vi "optimization_testing.vi"() -> (3 "Optimized Location":dbl[](array[numeric]), 10 "yStart":dbl=123.0 format="%#_13g", 11 "xStart":dbl=264.0 format="%#_13g")   [LabVIEW 2024]
uses:
  <vilib>/numeric/Random Number (Range) DBL.vi
  0b4b40c4-ef97-49a3-bff4-9c7e9883bc37.vi
  5b59031f-b1ff-41af-80a7-e72a33ebffa1.vi
  <vilib>/Array/Sort 2D Array - Pop Stack.vi
  <vilib>/Array/Sort 2D Array - Push Stack.vi
  0b4b40c4-ef97-49a3-bff4-9c7e9883bc37.vi/269d4b3b-47f5-49e3-8884-44851e4dd9d5.vi
  0b4b40c4-ef97-49a3-bff4-9c7e9883bc37.vi/6d99389c-673d-4efb-bf33-19b32bcf4cf8.vi
  5b59031f-b1ff-41af-80a7-e72a33ebffa1.vi/269d4b3b-47f5-49e3-8884-44851e4dd9d5.vi
  5b59031f-b1ff-41af-80a7-e72a33ebffa1.vi/6d99389c-673d-4efb-bf33-19b32bcf4cf8.vi
  <vilib>/Analysis/NI_AALBase.lvlib
panel:
  out "Array":dbl[](array[numeric])
  out "elapsed time (s)":dbl
  out "n":i32(slide) scale=0.0..1.0
  out "GrAsc - avgs":dbl[][](array[numeric])
  out "NM - avgs":dbl[][](array[numeric])
  in  "nTrials":i32=1000
  out "std dev of simplex values 2":dbl
  out "simplex leg lengths 2":dbl[](array[numeric])
  out "iterations timeout 2":bool
  out "simplex converge 2":bool
  out "value converge 2":bool
  out "Starting Points":dbl[][][](array[numeric])
  in  "k":dbl=50.0
  out "GrAsc res":dbl[](array[numeric])
  out "x_c":dbl[](array[numeric])
  out "x_e":dbl[](array[numeric])
  out "x_r":dbl[](array[numeric])
  out "x_o":dbl[](array[numeric])
  out "iterations timeout":bool
  out "simplex converge":bool
  out "value converge":bool
  out "simplex leg lengths":dbl[](array[numeric])
  out "std dev of simplex values":dbl
  in  "stop":bool
  # "Avg"
  # "Std Dev"
  # "X"
  # "Y"
  # "Value"
  # "n Trials"
  # "Failures"
  # "Avg"
  # "Std Dev"
  # "X"
  # "Y"
  # "Value"
  # "n Trials"
  # "Failures"
  # "centroid"
  # "reflection point"
  # "expansion point"
  # "contraction point"
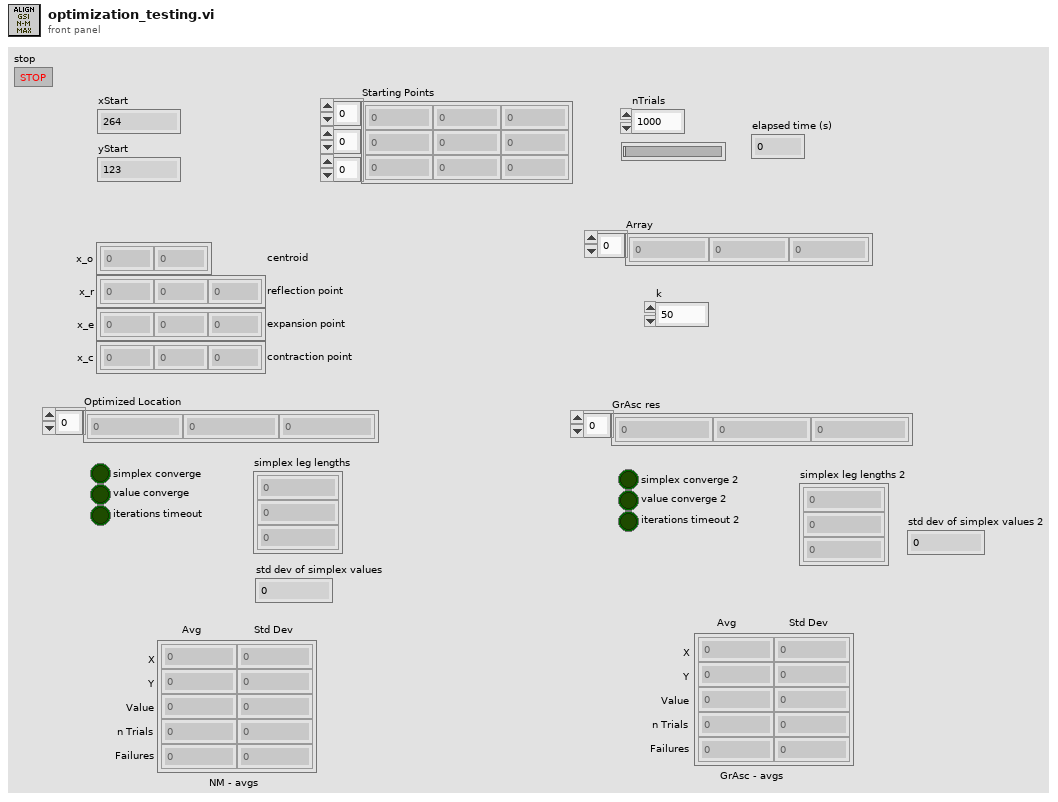
[diagram p1: front panel]
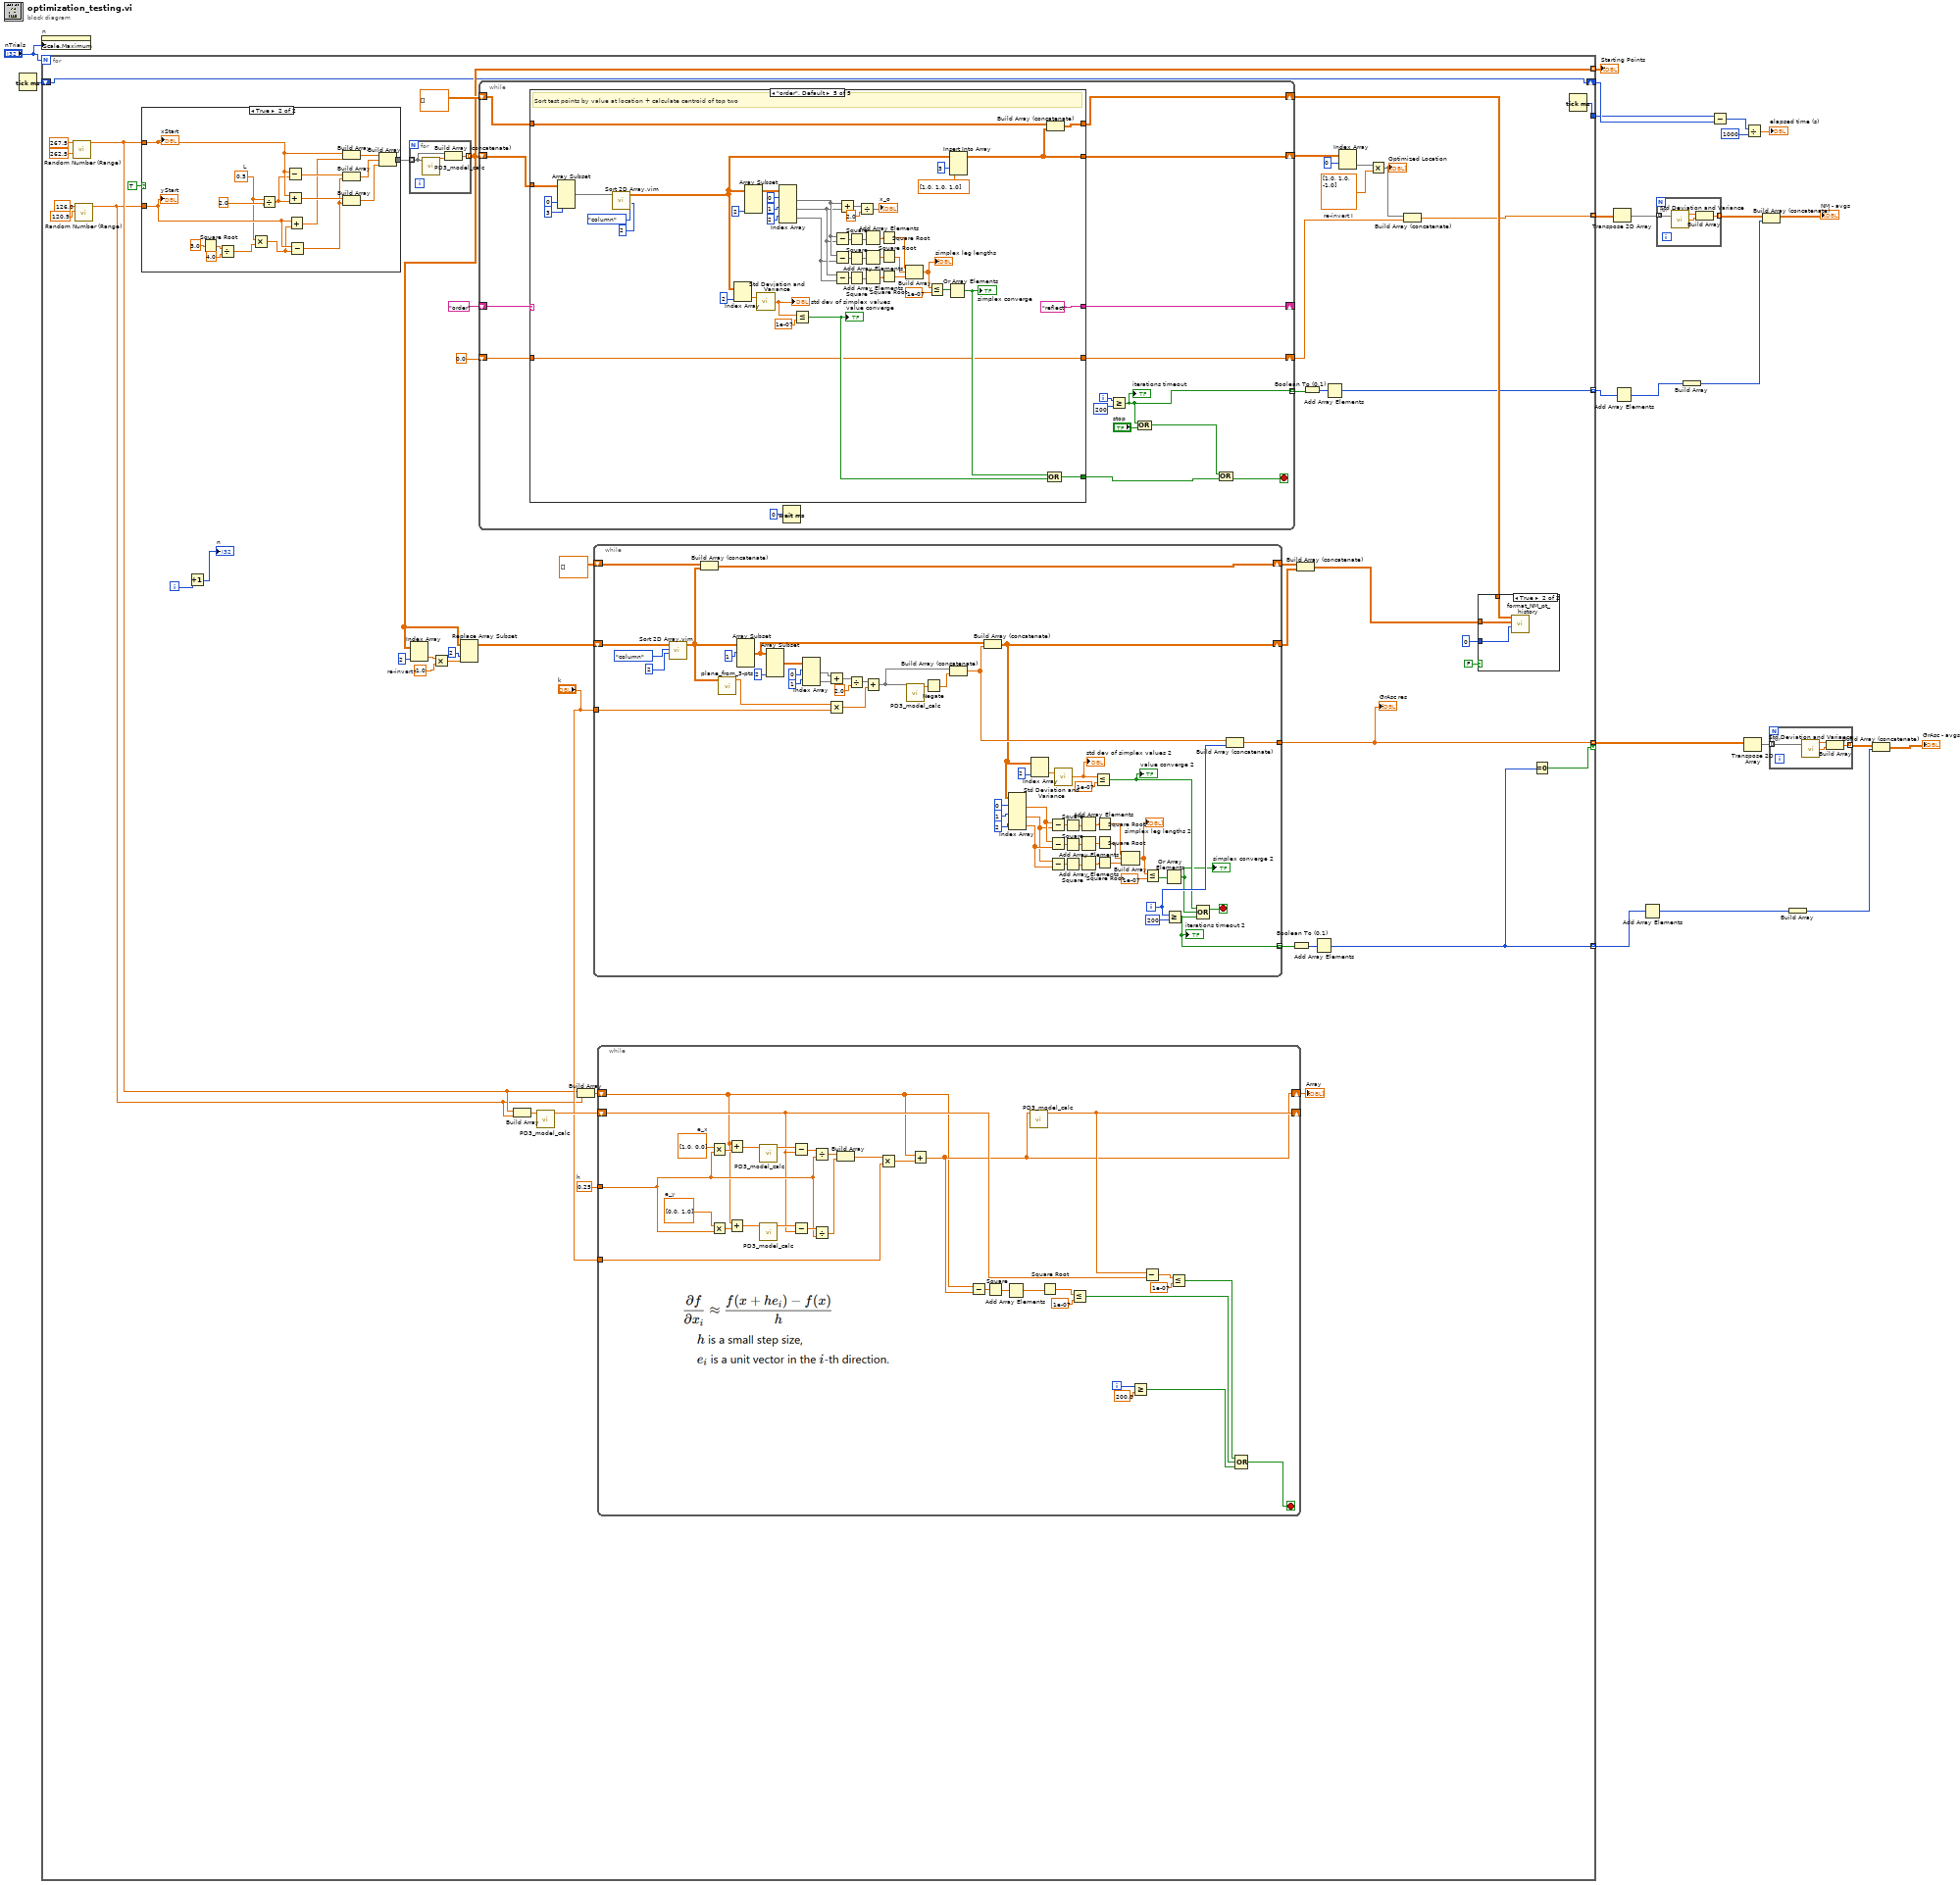
[diagram p0: block diagram]
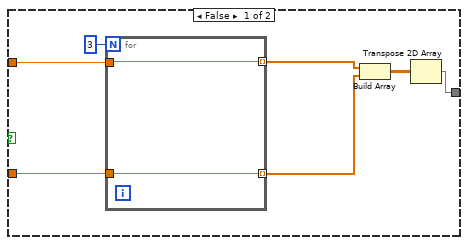
[diagram p3: hidden frame]
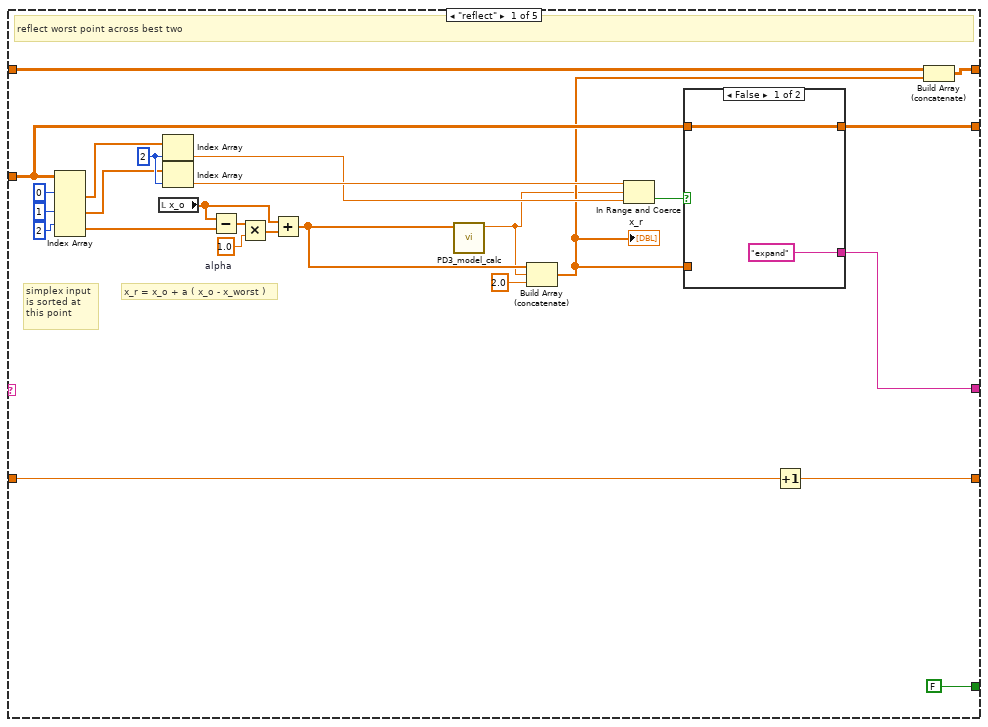
[diagram p4: hidden frame]
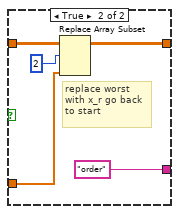
[diagram p5: hidden frame]
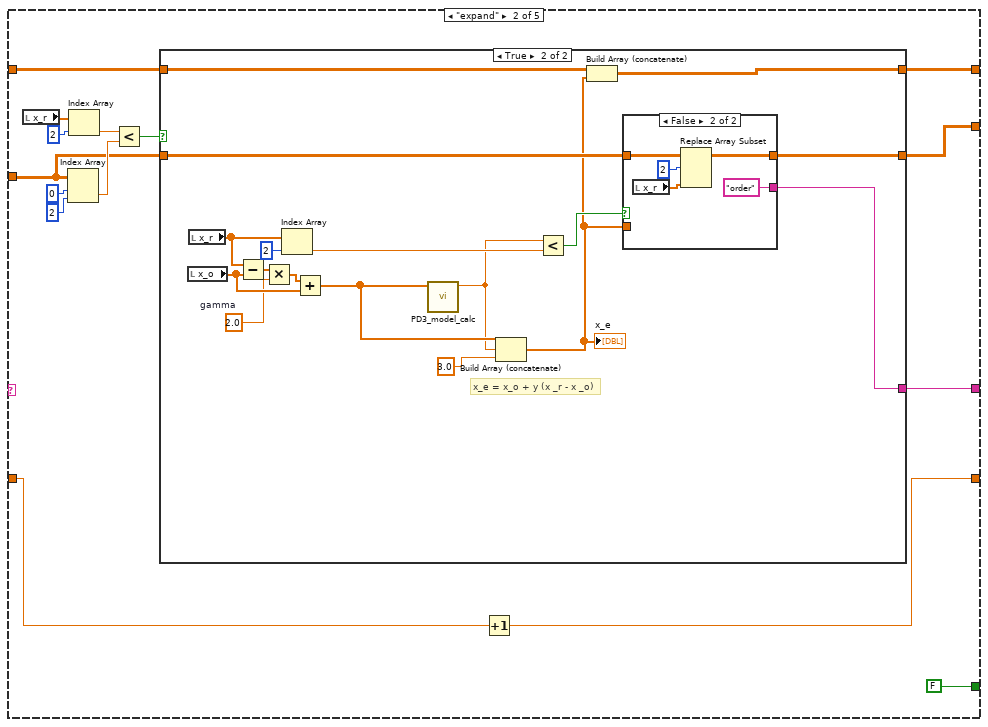
[diagram p6: hidden frame]
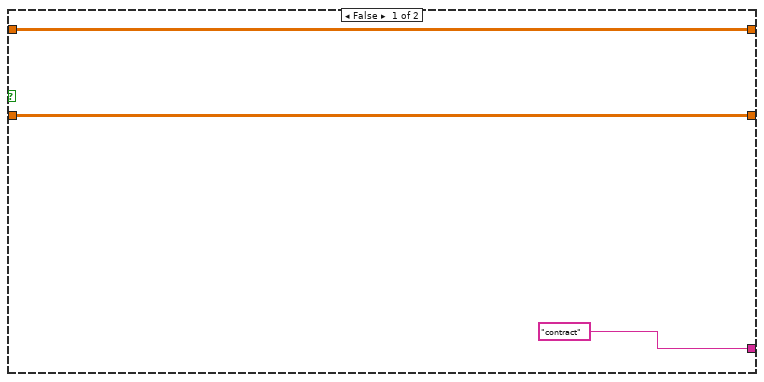
[diagram p7: hidden frame]
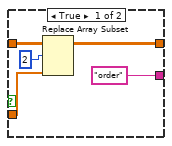
[diagram p8: hidden frame]
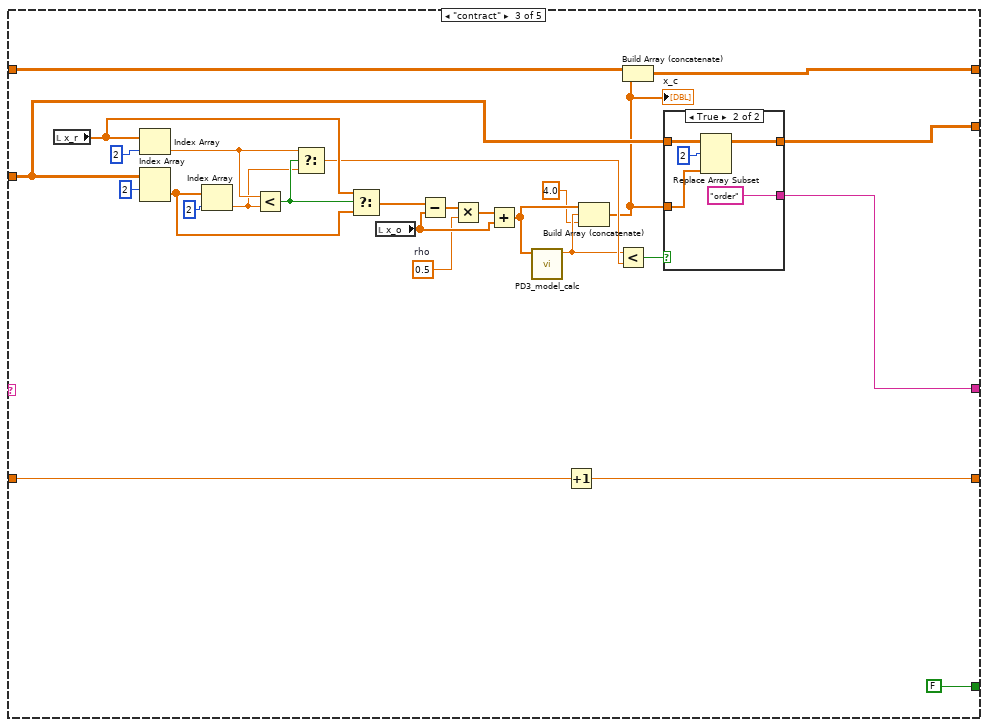
[diagram p9: hidden frame]
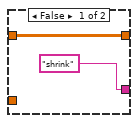
[diagram p10: hidden frame]
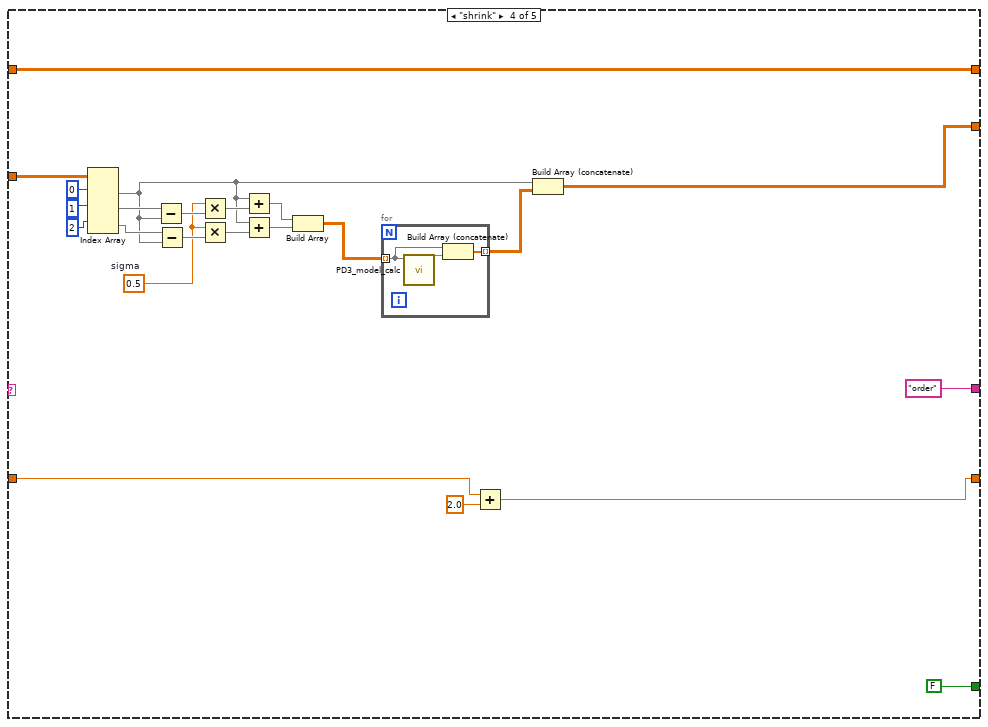
[diagram p11: hidden frame]
diagram:
  n1 = Tick Count (ms)() -> (millisecond timer value=w4:u32)
  n2 = property on="n" class="Slide (strict)"("Scale.Maximum"="nTrials") -> ()  [unwired: 2 in, 2 out]
  n3 = for {
    N: "nTrials" -> [_]
    tunnel: [w47] -> w21 mode=indexing
    tunnel: [w45] -> w20 mode=indexing
    tunnel: [w42] -> w15 mode=indexing if=w39
    tunnel: [w38] -> w14 mode=indexing
    tunnel: [w35] -> w10 mode=indexing
    shift-right: [w32] -> w3
    shift-left: w4 -> [w32]
    tunnel: [w31] -> w1
    i -> [w34]
    w28 = 0.25  # h
    w60 = -1.0  # re-invert I
    w67 = dbl[] [1.0, 1.0, -1.0]  # re-invert I
    n4 = call-poly <vilib>:"Random Number (Range).vi"("lower bound (0)"=262.5, "upper bound (100)"=267.5) -> ("number"=w26:dbl)  [unwired: 9 in]
    n5 = call-poly <vilib>:"Random Number (Range).vi"("lower bound (0)"=120.9 ("upper bound (100)"), "upper bound (100)"=126.0 ("lower bound (0)")) -> ("number"=w25:dbl)  [unwired: 9 in]
    n6 = case shown="True" TRUE {
      tunnel: [w109 w132] -> w55
      tunnel: w26 -> [w114 w124]
      tunnel: w25 -> [w113 w123]
      frame False {
        n7 = for {
          N: 3 -> [_]
          tunnel: w114 -> [w117]
          tunnel: [w117] -> w112 mode=indexing
          tunnel: w113 -> [w116]
          tunnel: [w116] -> w110 mode=indexing
        }
        n8 = Build Array(w112, w110) -> (w111:dbl[][])
        n9 = Transpose 2D Array(2D array=w111) -> (transposed array=w109:dbl[][])
      }
      frame True {
        w118 = 0.5  # L
        n10 = Square Root(x=3.0) -> (sqrt(x)=w131:dbl)
        n11 = Divide(x=w131, y=4.0) -> (x/y=w120:dbl)
        n12 = Multiply(x=w118, y=w120) -> (x*y=w119:dbl)
        n13 = Divide(x=w118, y=2.0) -> (x/y=w121:dbl)
        n14 = Subtract(x=w124, y=w121) -> (x-y=w128:dbl)
        n15 = Add(x=w124, y=w121) -> (x+y=w127:dbl)
        n16 = Add(x=w123, y=w119) -> (x+y=w126:dbl)
        n17 = Subtract(x=w123, y=w119) -> (x-y=w125:dbl)
        n18 = Build Array(w124, w126) -> (w133:dbl[])
        n19 = Build Array(w128, w125) -> (w134:dbl[])
        n20 = Build Array(w127, w125) -> (w135:dbl[])
        n21 = Build Array(w133, w134, w135) -> (w132:dbl[][])
        "xStart" <- w124
        "yStart" <- w123
      }
    }
    n22 = Increment(x=w34) -> (x+1=→"n":i32)
    n23 = for {
      tunnel: w55 -> [w193] mode=indexing
      tunnel: [w195] -> w47 mode=indexing
      n24 = call "PD3_model_calc.vi"("pos_in"=w193) -> ("I_out"=w194:dbl)  [unwired: 10 in]
      n25 = Build Array (concatenate)(w193, w194) -> (w195:dbl[])
    }
    n26 = Index Array(array=w47, index (col)=2 ("disabled index (col)")) -> (element=w58:dbl[])  [unwired: 1 in]
    n27 = Multiply(x=w58, y=w60) -> (x*y=w56:dbl[])
    n28 = Replace Array Subset(array=w47, new element=w56, index (col)=2 ("disabled index (col)")) -> (w54:dbl[][])  [unwired: 1 in]
    n29 = while {
      shift-right: [w209] -> w72
      shift-left: w47 -> [w207]
      shift-right: [w210] -> _
      shift-left: "order" -> [w211]
      shift-right: [w205] -> w66
      shift-left: dbl[][] [] -> [w206]
      shift-right: [w199] -> w43
      shift-left: 0.0 -> [w200]
      tunnel: [w198] -> w36 mode=indexing
      i -> [w201]
      stop <- w197 stop-if-true
      n30 = case shown="\"order\", Default" w211 {
        tunnel: w207 -> [w222 w252 w302 w345 w388]
        tunnel: [FALSE FALSE FALSE FALSE w364] -> w203
        tunnel: [w221 w251 w303 w334 w353] -> w209
        tunnel: [w223 w250 w304 "order" "reflect"] -> w210
        tunnel: w206 -> [w219 w248 w298 w332 w352]
        tunnel: [w218 w247 w295 w332 w358] -> w205
        tunnel: w200 -> [w213 w246 w291 w326 w350]
        tunnel: [w212 w245 w290 w325 w350] -> w199
        frame "reflect" {
          w214 = 1.0  # alpha
          w231 = 2 ("index")
          # "simplex input\nis sorted at\nthis point"
          # "x_r = x_o + a ( x_o - x_worst )"
          # "reflect worst point across best two"
          n31 = Index Array(array=w222, index (row) #1=0 ("index (row)"), index (row) #2=1 ("index (row)"), index (row) #3=2 ("index (row)")) -> (element #1=w230:dbl[], element #2=w229:dbl[], element #3=w232:dbl[])  [unwired: 3 in]
          n32 = local read "x_o"() -> (w224:dbl[])
          n33 = Index Array(array=w230, index=w231) -> (element=w227:dbl)
          n34 = Index Array(array=w229, index=w231) -> (element=w228:dbl)
          n35 = Subtract(x=w224, y=w232) -> (x-y=w236:dbl[])
          n36 = Multiply(x=w236, y=w214) -> (x*y=w235:dbl[])
          n37 = Add(x=w224, y=w235) -> (x+y=w225:dbl[])
          n38 = call "PD3_model_calc.vi"("pos_in"=w225) -> ("I_out"=w216:dbl)  [unwired: 10 in]
          n39 = Build Array (concatenate)(w225, w216, 2.0) -> (w217:dbl[])
          "x_r" <- w217
          n40 = In Range and Coerce(upper limit=w228, x=w216, lower limit=w227) -> (In Range?=w226:bool)  [unwired: 1 out]
          n41 = case shown="False" w226 {
            tunnel: ["expand" "order"] -> w223
            tunnel: w222 -> [w238 w244]
            tunnel: [w238 w241] -> w221
            tunnel: w217 -> [_ w242]
            frame False {
            }
            frame True {
              # "replace worst \nwith x_r go back\nto start"
              n42 = Replace Array Subset(array=w244, new element=w242, index (row)=2) -> (w241:dbl[][])  [unwired: 1 in]
            }
          }
          n43 = Increment(x=w213) -> (x+1=w212:dbl)
          n44 = Build Array (concatenate)(w219, w217) -> (w218:dbl[][])
        }
        frame "expand" {
          n45 = local read "x_r"() -> (w257:dbl[])
          n46 = Index Array(array=w252, index (row)=0, index (col)=2 ("disabled index (col)")) -> (element=w255:dbl)
          n47 = Index Array(array=w257, index=2) -> (element=w254:dbl)
          n48 = Less?(x=w254, y=w255) -> (x < y?=w253:bool)
          n49 = case shown="True" w253 {
            tunnel: w252 -> [w262 w272]
            tunnel: [w262 w270] -> w251
            tunnel: ["contract" w269] -> w250
            tunnel: w248 -> [w260 w267]
            tunnel: [w260 w266] -> w247
            frame False {
            }
            frame True {
              w263 = 2.0  # gamma
              # "x_e = x_o + y (x _r - x _o)"
              n50 = local read "x_o"() -> (w277:dbl[])
              n51 = local read "x_r"() -> (w276:dbl[])
              n52 = Subtract(x=w276, y=w277) -> (x-y=w279:dbl[])
              n53 = Multiply(x=w279, y=w263) -> (x*y=w278:dbl[])
              n54 = Index Array(array=w276, index=2) -> (element=w274:dbl)
              n55 = Add(x=w278, y=w277) -> (x+y=w271:dbl[])
              n56 = call "PD3_model_calc.vi"("pos_in"=w271) -> ("I_out"=w268:dbl)  [unwired: 10 in]
              n57 = Build Array (concatenate)(w271, w268, 3.0) -> (w265:dbl[])
              "x_e" <- w265
              n58 = Less?(x=w268, y=w274) -> (x < y?=w273:bool)
              n59 = Build Array (concatenate)(w267, w265) -> (w266:dbl[][])
              n60 = case shown="False" w273 {
                tunnel: w272 -> [w283 w288]
                tunnel: w265 -> [w282 _]
                tunnel: [w281 w287] -> w270
                tunnel: ["order" "order"] -> w269
                frame True {
                  n61 = Replace Array Subset(array=w283, new element=w282, index (row)=2) -> (w281:dbl[][])  [unwired: 1 in]
                }
                frame False {
                  n62 = local read "x_r"() -> (w285:dbl[])
                  n63 = Replace Array Subset(array=w288, new element=w285, index (row)=2) -> (w287:dbl[][])  [unwired: 1 in]
                }
              }
            }
          }
          n64 = Increment(x=w246) -> (x+1=w245:dbl)
        }
        frame "contract" {
          w292 = 0.5  # rho
          n65 = local read "x_r"() -> (w313:dbl[])
          n66 = Index Array(array=w313, index=2) -> (element=w308:dbl)
          n67 = Index Array(array=w302, index (row)=2) -> (element=w312:dbl[])  [unwired: 1 in]
          n68 = Index Array(array=w312, index=2) -> (element=w307:dbl)
          n69 = Less?(x=w308, y=w307) -> (x < y?=w309:bool)
          n70 = Select(t=w308, s=w309, f=w307) -> (s? t:f=w306:dbl)
          n71 = Select(t=w313, s=w309, f=w312) -> (s? t:f=w311:dbl[])
          n72 = local read "x_o"() -> (w300:dbl[])
          n73 = Subtract(x=w311, y=w300) -> (x-y=w310:dbl[])
          n74 = Multiply(x=w310, y=w292) -> (x*y=w301:dbl[])
          n75 = Add(x=w301, y=w300) -> (x+y=w297:dbl[])
          n76 = call "PD3_model_calc.vi"("pos_in"=w297) -> ("I_out"=w296:dbl)  [unwired: 10 in]
          n77 = Increment(x=w291) -> (x+1=w290:dbl)
          n78 = Build Array (concatenate)(w297, w296, 4.0 ("array")) -> (w294:dbl[])
          "x_c" <- w294
          n79 = Less?(x=w296, y=w306) -> (x < y?=w305:bool)
          n80 = Build Array (concatenate)(w298, w294) -> (w295:dbl[][])
          n81 = case shown="True" w305 {
            tunnel: ["shrink" "order"] -> w304
            tunnel: [w317 w319] -> w303
            tunnel: w302 -> [w317 w321]
            tunnel: w294 -> [_ w320]
            frame False {
            }
            frame True {
              n82 = Replace Array Subset(array=w321, new element=w320, index (row)=2) -> (w319:dbl[][])  [unwired: 1 in]
            }
          }
        }
        frame "shrink" {
          w331 = 0.5  # sigma
          n83 = Index Array(array=w345, index (row) #1=0 ("index (row)"), index (row) #2=1 ("index (row)"), index (row) #3=2 ("index (row)")) -> (element #1=w335:dbl[], element #2=w341:dbl[], element #3=w340:dbl[])  [unwired: 3 in]
          n84 = Subtract(x=w341, y=w335) -> (x-y=w338:dbl[])
          n85 = Subtract(x=w340, y=w335) -> (x-y=w339:dbl[])
          n86 = Multiply(x=w331, y=w338) -> (x*y=w337:dbl[])
          n87 = Multiply(x=w331, y=w339) -> (x*y=w336:dbl[])
          n88 = Add(x=w335, y=w337) -> (x+y=w330:dbl[])
          n89 = Add(x=w335, y=w336) -> (x+y=w329:dbl[])
          n90 = Build Array(w330, w329) -> (w328:dbl[][])
          n91 = for {
            tunnel: w328 -> [w347] mode=indexing
            tunnel: [w349] -> w327 mode=indexing
            n92 = call "PD3_model_calc.vi"("pos_in"=w347) -> ("I_out"=w348:dbl)  [unwired: 10 in]
            n93 = Build Array (concatenate)(w347, w348) -> (w349:dbl[])
          }
          n94 = Add(x=w326, y=2.0) -> (x+y=w325:dbl)
          n95 = Build Array (concatenate)(w335, w327) -> (w334:dbl[][])
        }
        frame "order", Default {
          # "Sort test points by value at location + calculate centroid of top two"
          n96 = Array Subset(array=w388, index (col)=0 ("index"), length (col)=3 ("length")) -> (w351:dbl[][])  [unwired: 2 in]
          n97 = call "Sort 2D Array.vim"("index"=2, "dimension to index (column)"=enum16{"column", "row"}."column", "2D array"=w351) -> ("sorted 2D array"=w356:dbl[][])  [unwired: 7 in, 1 out]
          n98 = Index Array(array=w356, index (col)=2 ("index")) -> (element=w382:dbl[])  [unwired: 1 in]
          n99 = Array Subset(array=w356, length (col)=2 ("length")) -> (w381:dbl[][])  [unwired: 3 in]
          n100 = call <vilib>:"Std Deviation and Variance.vi"("X"=w382) -> ("standard deviation"=w357:dbl)  [unwired: 1 in, 2 out]
          "std dev of simplex values" <- w357
          n101 = Index Array(array=w381, index (row) #1=0 ("index (row)"), index (row) #2=1 ("index (row)"), index (row) #3=2 ("index (row)")) -> (element #1=w361:dbl[], element #2=w360:dbl[], element #3=w359:dbl[])  [unwired: 3 in]
          n102 = Less Or Equal?(x=w357, y=1e-07) -> (x <= y?=w363:bool)
          "value converge" <- w363
          n103 = Subtract(x=w361, y=w360) -> (x-y=w379:dbl[])
          n104 = Subtract(x=w361, y=w359) -> (x-y=w371:dbl[])
          n105 = Subtract(x=w360, y=w359) -> (x-y=w374:dbl[])
          n106 = Add(x=w361, y=w360) -> (x+y=w386:dbl[])
          n107 = Square(x=w379) -> (x^2=w378:dbl[])
          n108 = Square(x=w371) -> (x^2=w375:dbl[])
          n109 = Square(x=w374) -> (x^2=w373:dbl[])
          n110 = Divide(x=w386, y=2.0) -> (x/y=→"x_o":dbl[])
          n111 = Add Array Elements(numeric array=w378) -> (sum=w377:dbl)
          n112 = Add Array Elements(numeric array=w375) -> (sum=w376:dbl)
          n113 = Add Array Elements(numeric array=w373) -> (sum=w372:dbl)
          n114 = Square Root(x=w377) -> (sqrt(x)=w368:dbl)
          n115 = Square Root(x=w376) -> (sqrt(x)=w369:dbl)
          n116 = Square Root(x=w372) -> (sqrt(x)=w370:dbl)
          n117 = Build Array(w368, w369, w370) -> (w367:dbl[])
          "simplex leg lengths" <- w367
          n118 = Less Or Equal?(x=w367, y=1e-07) -> (x <= y?=w365:bool[])
          n119 = Or Array Elements(Boolean array=w365) -> (logical OR=w362:bool)
          "simplex converge" <- w362
          n120 = Insert Into Array(array=w356, index (col)=3 ("disabled index (col)"), new element=dbl[] [1.0, 1.0, 1.0] ("new element/subarray")) -> (w353:dbl[][])  [unwired: 1 in]
          n121 = Build Array (concatenate)(w352, w353) -> (w358:dbl[][])
          n122 = Compound Arithmetic op=OR(w362, w363) -> (w364:bool)
        }
      }
      n123 = Wait (ms)(milliseconds to wait=u32 0) -> ()  [unwired: 1 out]
      n124 = Greater Or Equal?(x=w201, y=200) -> (x >= y?=w198:bool)
      "iterations timeout" <- w198
      n125 = Compound Arithmetic op=OR(w198, "stop") -> (w196:bool)
      n126 = Compound Arithmetic op=OR(w196, w203) -> (w197:bool)
    }
    n127 = Build Array(w26, w25) -> (w30:dbl[])
    n128 = call "PD3_model_calc.vi"("pos_in"=w30) -> ("I_out"=w29:dbl)  [unwired: 10 in]
    n129 = Build Array(w26, w25) -> (w24:dbl[])
    n130 = while {
      tunnel: "k" -> [w168]
      shift-right: [w171] -> w53
      shift-left: dbl[][] [] -> [w192]
      shift-right: [w149] -> w52
      shift-left: w54 -> [w189]
      tunnel: [w163] -> w42
      tunnel: [w136] -> w41 mode=indexing
      i -> [w162]
      stop <- w164 stop-if-true
      n131 = call "Sort 2D Array.vim"("index"=2, "dimension to index (column)"=enum16{"column", "row"}."column", "2D array"=w189) -> ("sorted 2D array"=w170:dbl[][])  [unwired: 7 in, 1 out]
      n132 = Build Array (concatenate)(w192, w170) -> (w171:dbl[][])
      n133 = call "plane_from_3-pts.vi"("Input"=w170) -> ("gradient-out"=w173:dbl[])  [unwired: 9 in, 1 out]
      n134 = Array Subset(array=w170, index (row)=1 ("index")) -> (w178:dbl[][])  [unwired: 3 in]
      n135 = Array Subset(array=w178, length (col)=2 ("length")) -> (w180:dbl[][])  [unwired: 3 in]
      n136 = Index Array(array=w180, index (row) #1=0 ("index (row)"), index (row) #2=1 ("index (row)")) -> (element #1=w185:dbl[], element #2=w184:dbl[])  [unwired: 2 in]
      n137 = Add(x=w185, y=w184) -> (x+y=w183:dbl[])
      n138 = Multiply(x=w173, y=w168) -> (x*y=w174:dbl[])
      n139 = Divide(x=w183, y=2.0) -> (x/y=w176:dbl[])
      n140 = Add(x=w176, y=w174) -> (x+y=w175:dbl[])
      n141 = call "PD3_model_calc.vi"("pos_in"=w175) -> ("I_out"=w179:dbl)  [unwired: 10 in]
      n142 = Negate(x=w179) -> (-x=w177:dbl)
      n143 = Build Array (concatenate)(w175, w177) -> (w169:dbl[])
      n144 = Build Array (concatenate)(w178, w169) -> (w149:dbl[][])
      n145 = Index Array(array=w149, index (row) #1=0 ("index (row)"), index (row) #2=1 ("index (row)"), index (row) #3=2 ("index (row)")) -> (element #1=w148:dbl[], element #2=w146:dbl[], element #3=w147:dbl[])  [unwired: 3 in]
      n146 = Index Array(array=w149, index (col)=2 ("index")) -> (element=w167:dbl[])  [unwired: 1 in]
      n147 = Subtract(x=w148, y=w146) -> (x-y=w150:dbl[])
      n148 = Subtract(x=w148, y=w147) -> (x-y=w158:dbl[])
      n149 = Subtract(x=w146, y=w147) -> (x-y=w155:dbl[])
      n150 = call <vilib>:"Std Deviation and Variance.vi"("X"=w167) -> ("standard deviation"=w137:dbl)  [unwired: 1 in, 2 out]
      "std dev of simplex values 2" <- w137
      n151 = Square(x=w150) -> (x^2=w151:dbl[])
      n152 = Square(x=w158) -> (x^2=w154:dbl[])
      n153 = Square(x=w155) -> (x^2=w156:dbl[])
      n154 = Add Array Elements(numeric array=w151) -> (sum=w152:dbl)
      n155 = Add Array Elements(numeric array=w154) -> (sum=w153:dbl)
      n156 = Add Array Elements(numeric array=w156) -> (sum=w157:dbl)
      n157 = Less Or Equal?(x=w137, y=1e-07) -> (x <= y?=w140:bool)
      "value converge 2" <- w140
      n158 = Square Root(x=w152) -> (sqrt(x)=w161:dbl)
      n159 = Square Root(x=w153) -> (sqrt(x)=w160:dbl)
      n160 = Square Root(x=w157) -> (sqrt(x)=w159:dbl)
      n161 = Build Array(w161, w160, w159) -> (w138:dbl[])
      "simplex leg lengths 2" <- w138
      n162 = Less Or Equal?(x=w138, y=1e-07) -> (x <= y?=w144:bool[])
      n163 = Or Array Elements(Boolean array=w144) -> (logical OR=w139:bool)
      "simplex converge 2" <- w139
      n164 = Greater Or Equal?(x=w162, y=200) -> (x >= y?=w136:bool)
      "iterations timeout 2" <- w136
      n165 = Compound Arithmetic op=OR(w140, w139, w136) -> (w164:bool)
      n166 = Build Array (concatenate)(w169, w162) -> (w163:dbl[])
    }
    "GrAsc res" <- w42
    n167 = while {
      tunnel: w28 -> [w95]
      tunnel: "k" -> [w91]
      shift-right: [w87] -> w23
      shift-left: w24 -> [w73]
      shift-right: [w89] -> _
      shift-left: w29 -> [w88]
      i -> [w78]
      stop <- w77 stop-if-true
      w96 = dbl[] [0.0, 1.0]  # e_y
      w105 = dbl[] [1.0, 0.0]  # e_x
      n168 = Multiply(x=w105, y=w95) -> (x*y=w104:dbl[])
      n169 = Multiply(x=w96, y=w95) -> (x*y=w97:dbl[])
      n170 = Add(x=w73, y=w104) -> (x+y=w103:dbl[])
      n171 = Add(x=w73, y=w97) -> (x+y=w98:dbl[])
      n172 = call "PD3_model_calc.vi"("pos_in"=w103) -> ("I_out"=w102:dbl)  [unwired: 10 in]
      n173 = call "PD3_model_calc.vi"("pos_in"=w98) -> ("I_out"=w99:dbl)  [unwired: 10 in]
      n174 = Subtract(x=w102, y=w88) -> (x-y=w101:dbl)
      n175 = Subtract(x=w99, y=w88) -> (x-y=w100:dbl)
      n176 = Divide(x=w101, y=w95) -> (x/y=w94:dbl)
      n177 = Divide(x=w100, y=w95) -> (x/y=w93:dbl)
      n178 = Build Array(w94, w93) -> (w92:dbl[])
      n179 = Multiply(x=w92, y=w91) -> (x*y=w90:dbl[])
      n180 = Add(x=w73, y=w90) -> (x+y=w87:dbl[])
      n181 = Subtract(x=w73, y=w87) -> (x-y=w86:dbl[])
      n182 = Square(x=w86) -> (x^2=w85:dbl[])
      n183 = Add Array Elements(numeric array=w85) -> (sum=w84:dbl)
      n184 = call "PD3_model_calc.vi"("pos_in"=w87) -> ("I_out"=w89:dbl)  [unwired: 10 in]
      n185 = Square Root(x=w84) -> (sqrt(x)=w80:dbl)
      n186 = Less Or Equal?(x=w80, y=1e-07) -> (x <= y?=w75:bool)
      n187 = Greater Or Equal?(x=w78, y=200.0) -> (x >= y?=w74:bool)
      n188 = Subtract(x=w89, y=w88) -> (x-y=w82:dbl)
      n189 = Less Or Equal?(x=w82, y=1e-07) -> (x <= y?=w76:bool)
      n190 = Compound Arithmetic op=OR(w76, w75, w74) -> (w77:bool)
    }
    "Array" <- w23
    n191 = Boolean To (0,1)(Boolean=w41) -> (0, 1=w40:i16[])
    n192 = Build Array (concatenate)(w53, w52) -> (w50:dbl[][])
    n193 = Boolean To (0,1)(Boolean=w36) -> (0, 1=w37:i16[])
    n194 = Add Array Elements(numeric array=w40) -> (sum=w38:i16)
    n195 = Add Array Elements(numeric array=w37) -> (sum=w35:i16)
    n196 = Index Array(array=w72, index (row)=0) -> (element=w68:dbl[])  [unwired: 1 in]
    n197 = Multiply(x=w68, y=w67) -> (x*y=w46:dbl[])
    "Optimized Location" <- w46
    n198 = Build Array (concatenate)(w46, w43) -> (w45:dbl[])
    n199 = case shown="True" FALSE {
      tunnel: w66 -> [_ w108]
      tunnel: w50 -> [_ w107]
      tunnel: 0 ("trial #") -> [_ w106]
      frame False {
      }
      frame True {
        n200 = call "format_NM_pt_history.vi"("trial #"=w106, "GrAsc in"=w107, "NM in"=w108) -> ()  [unwired: 9 in]
      }
    }
    n201 = Equal To 0?(x=w38) -> (x = 0?=w39:bool)
    n202 = Tick Count (ms)() -> (millisecond timer value=w31:u32)
  }
  "Starting Points" <- w21
  n203 = Transpose 2D Array(2D array=w20) -> (transposed array=w19:dbl[][])
  n204 = Add Array Elements(numeric array=w10) -> (sum=w11:i16)
  n205 = Add Array Elements(numeric array=w14) -> (sum=w13:i16)
  n206 = for {
    tunnel: w19 -> [w400] mode=indexing
    tunnel: [w397] -> w18 mode=indexing
    n207 = call <vilib>:"Std Deviation and Variance.vi"("X"=w400) -> ("mean"=w399:dbl, "standard deviation"=w398:dbl)  [unwired: 1 in, 1 out]
    n208 = Build Array(w399, w398) -> (w397:dbl[])
  }
  n209 = Build Array(w11) -> (w8:i16[])
  n210 = Subtract(x=w1, y=w3) -> (x-y=w6:u32)
  n211 = Transpose 2D Array(2D array=w15) -> (transposed array=w16:dbl[][])
  n212 = Divide(x=w6, y=u32 1000) -> (x/y=→"elapsed time (s)":dbl)
  n213 = Build Array (concatenate)(w18, w8) -> (→"NM - avgs":dbl[][])
  n214 = for {
    tunnel: w16 -> [w401] mode=indexing
    tunnel: [w402] -> w17 mode=indexing
    n215 = call <vilib>:"Std Deviation and Variance.vi"("X"=w401) -> ("mean"=w404:dbl, "standard deviation"=w403:dbl)  [unwired: 1 in, 1 out]
    n216 = Build Array(w404, w403) -> (w402:dbl[])
  }
  n217 = Build Array(w13) -> (w12:i16[])
  n218 = Build Array (concatenate)(w17, w12) -> (→"GrAsc - avgs":dbl[][])
